vi "test Deployment Switch and RaF Diff Resource.vi"(8 "error in (no error)":errorcluster, 11 "TestCase in":refnum<class "Routing and Faulting System Tests.lvclass">) -> (0 "error out":errorcluster, 3 "TestCase out":refnum<class "Routing and Faulting System Tests.lvclass">)   [LabVIEW 2017, in "Routing and Faulting System Tests.lvclass"]
uses:
  Routing and Faulting System Tests.lvclass
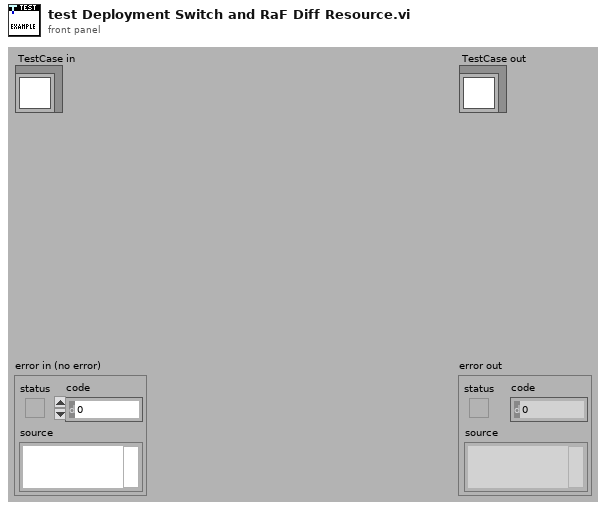
[diagram p1: front panel]
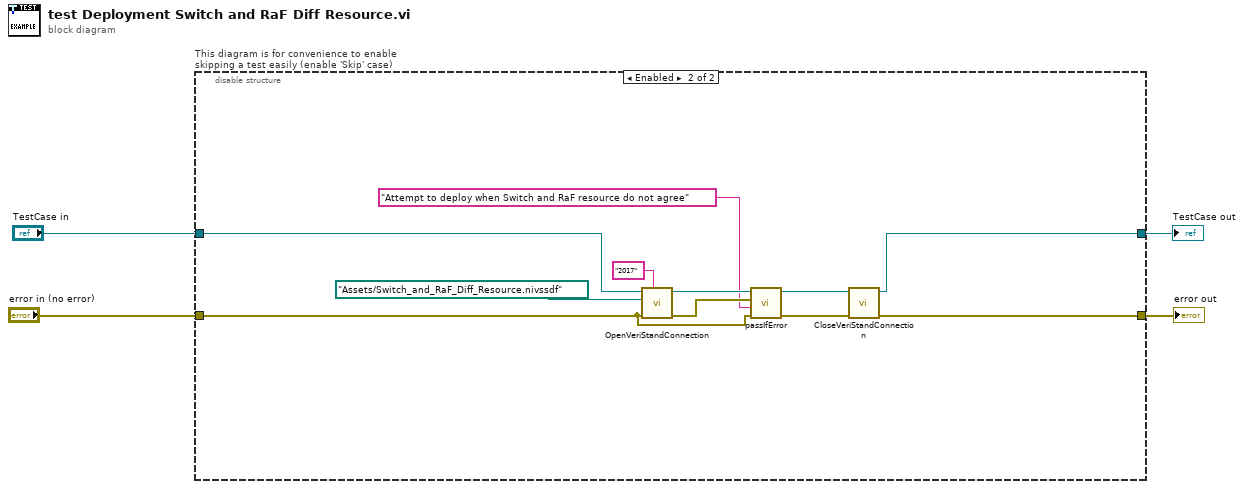
[diagram p0: block diagram]
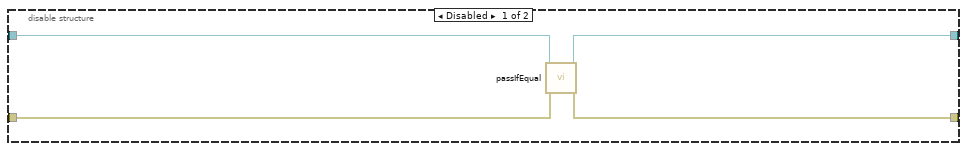
[diagram p2: hidden frame]
diagram:
  n1 = disable-structure "This diagram is for convenience to enable skipping a test easily (enable 'Skip' case)" shown="Enabled" {
    disable-tunnel: "TestCase in" -> [w8 w19]
    disable-tunnel: [w7 w18] -> w1
    disable-tunnel: [w6 w17] -> w3
    disable-tunnel: "error in (no error)" -> [w5 w9]
    frame Disabled {
      n2 = call-dynamic "passIfEqual.vi"("error in (no error)"=w5, "TestCase in"=w8) -> ("error out"=w6:errorcluster, "TestCase out"=w7:refnum<class "Routing and Faulting System Tests.lvclass">)  [unwired: 8 in]
    }
    frame Enabled {
      n3 = call-dynamic "OpenVeriStandConnection.vi"("Minimum VeriStand Version (2015)"="2017", "error in (no error)"=w9, "System Definition File"=path "Assets/Switch_and_RaF_Diff_Resource.nivssdf", "VeriStand Test Case in"=w19) -> ("error out"=w12:errorcluster, "VeriStand Test Case out"=w14:refnum<class "Routing and Faulting System Tests.lvclass">)  [unwired: 5 in, 1 out]
      n4 = call-dynamic "passIfError.vi"("error in (no error)"=w9, "task (\"\")"="Attempt to deploy when Switch and RaF resource do not agree" ("task (\"\")"), "error"=w12, "TestCase in"=w14) -> ("error out"=w11:errorcluster, "TestCase out"=w13:refnum<class "Routing and Faulting System Tests.lvclass">)  [unwired: 6 in]
      n5 = call-dynamic "CloseVeriStandConnection.vi"("error in (no error)"=w11, "VeriStand Test Case in"=w13) -> ("error out"=w17:errorcluster, "VeriStand Test Case out"=w18:refnum<class "Routing and Faulting System Tests.lvclass">)  [unwired: 8 in]
    }
  }
  "error out" <- w3
  "TestCase out" <- w1
